vi "Set All CD Item Property Values.vi"(8 "error in (no error)":errorcluster, 11 "CD Parameter Manager in":refnum<class "CD Parameter Manager.lvclass">) -> (0 "error out":errorcluster, 3 "CD Parameter Manager out":refnum<class "CD Parameter Manager.lvclass">)   [LabVIEW 2016, in "CD Parameter Manager API.lvlib" / "CD Parameter Manager.lvclass"]
uses:
  CD Parameter Manager.lvclass
  Parameter Class/Parameter.lvclass
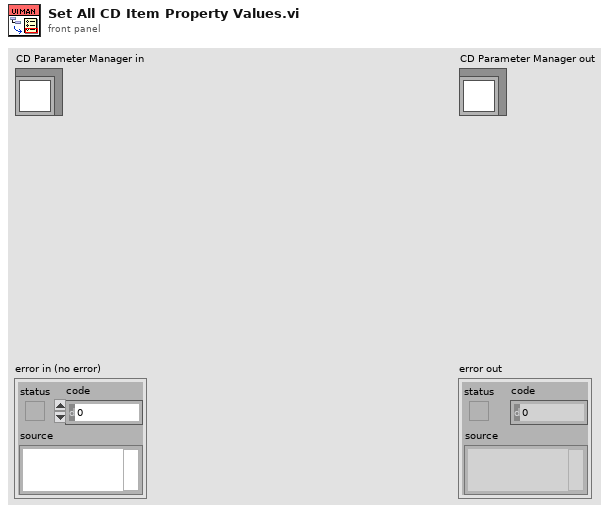
[diagram p1: front panel]
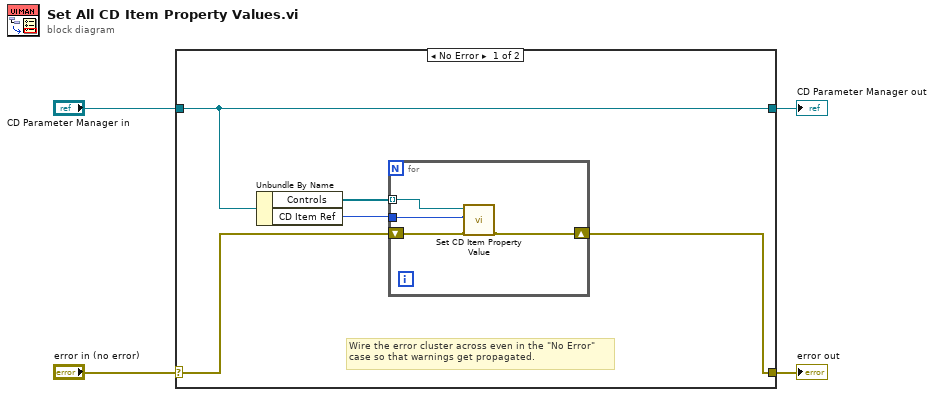
[diagram p0: block diagram]
diagram:
  n1 = case shown="No Error" "error in (no error)" {
    selector: "error in (no error)" -> [w6 w15]
    tunnel: [w5 w15] -> w3
    tunnel: [w7 w14] -> w1
    tunnel: "CD Parameter Manager in" -> [w7 w14]
    frame No Error {
      # "Wire the error cluster across even in the \"No Error\"\ncase so that warnings get propagated."
      n2 = Unbundle By Name(w7) -> ("Controls"=w9:refnum<class "Parameter.lvclass">[], "CD Item Ref"=w8:u64)
      n3 = for {
        tunnel: w8 -> [w11]
        tunnel: w9 -> [w10] mode=indexing
        shift-right: [w12] -> w5
        shift-left: w6 -> [w13]
        n4 = call-dynamic "Set CD Item Property Value.vi"("error in (no error)"=w13, "CD Item Ref in"=w11, "Parameter in"=w10) -> ("error out"=w12:errorcluster)  [unwired: 7 in, 1 out]
      }
    }
    frame Error {
    }
  }
  "error out" <- w3
  "CD Parameter Manager out" <- w1
